vi "get_opc.vi"(8 "error in (no error)":errorcluster, 11 "VISA Refnum in":refnum<visa-resource-name>) -> (0 "error out":errorcluster, 2 "OPC":string, 3 "VISA Refnum out":refnum<visa-resource-name>)   [LabVIEW 2018, in "Aim-TTi CPX400SP.lvlib"]
uses:
  <instrlib>/Aim-TTi CPX400SP/Aim-TTi CPX400SP.lvlib
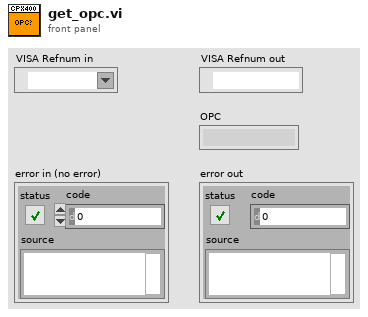
[diagram p1: front panel]
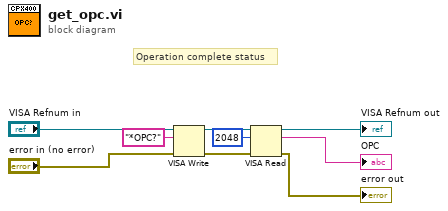
[diagram p0: block diagram]
diagram:
  # "Operation complete status"
  n1 = VISA Write(VISA resource name="VISA Refnum in", write buffer="*OPC?", error in (no error)="error in (no error)") -> (VISA resource name out=w1:refnum<visa-resource-name>, error out=w2:errorcluster)  [unwired: 1 out]
  n2 = VISA Read(VISA resource name=w1, byte count=u32 2048, error in (no error)=w2) -> (VISA resource name out=→"VISA Refnum out":refnum<visa-resource-name>, read buffer=→"OPC":string, error out=→"error out":errorcluster)  [unwired: 1 out]
